vi "GetPersonnelReportData.vi"(8 "error in":errorcluster, 9 "From":timestamp, 10 "To":timestamp, 11 "PersonnelName":string) -> (0 "error out":errorcluster, 2 "PersonnelReport":T1)   [LabVIEW 2015]
uses:
  TypeDef/PersonnelReport.ctl
  Database/DatabaseApi.lvlib
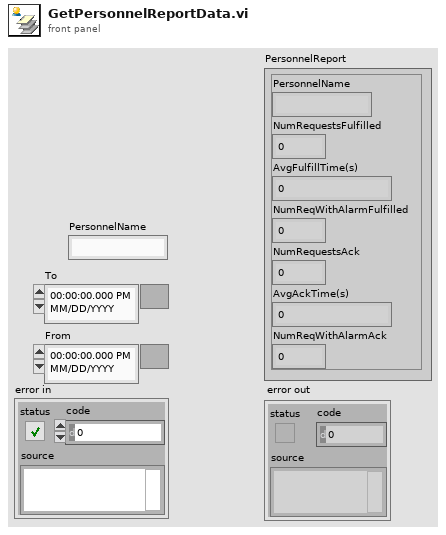
[diagram p1: front panel]
types:
  T1 = typedef "PersonnelReport.ctl" = cluster{"PersonnelName":string, "NumRequestsFulfilled":i32, "AvgFulfillTime(s)":dbl, "NumReqWithAlarmFulfilled":i32, "NumRequestsAck":i32, "AvgAckTime(s)":dbl, "NumReqWithAlarmAck":i32}
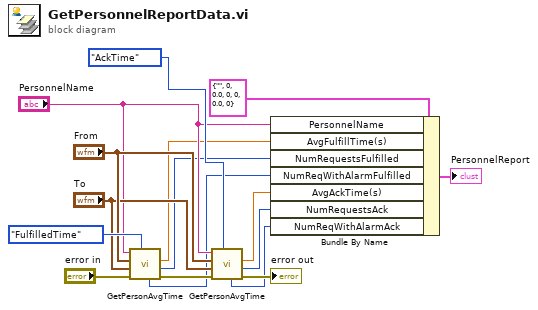
[diagram p0: block diagram]
diagram:
  n1 = call "GetPersonAvgTime.vi"("TimeToCheck"=enum16{"AckTime", "FulfilledTime"}."FulfilledTime", "error in"="error in", "To"="To", "From"="From", "PersonnelName"="PersonnelName") -> ("error out"=w15:errorcluster, "NumOfRequests"=w5:i32, "AvgTime(s)"=w4:dbl, "NumOfAlarms"=w6:i32)  [unwired: 3 in]
  n2 = call "GetPersonAvgTime.vi"("TimeToCheck"=enum16{"AckTime", "FulfilledTime"}."AckTime", "error in"=w15, "To"="To", "From"="From", "PersonnelName"="PersonnelName") -> ("error out"=→"error out":errorcluster, "NumOfRequests"=w2:i32, "AvgTime(s)"=w3:dbl, "NumOfAlarms"=w1:i32)  [unwired: 3 in]
  n3 = Bundle By Name(cluster=T1 {"PersonnelName"="", "NumRequestsFulfilled"=0, "AvgFulfillTime(s)"=0.0, "NumReqWithAlarmFulfilled"=0, "NumRequestsAck"=0, "AvgAckTime(s)"=0.0, "NumReqWithAlarmAck"=0} ("PersonnelReport"), "PersonnelName"="PersonnelName", "AvgFulfillTime(s)"=w4, "NumRequestsFulfilled"=w5, "NumReqWithAlarmFulfilled"=w6, "AvgAckTime(s)"=w3, "NumRequestsAck"=w2, "NumReqWithAlarmAck"=w1) -> (→"PersonnelReport":T1)
